vi "叶绿素a_获取温度和叶绿素值.vi"(8 "error in (no error)":errorcluster caption="错误输入（无错误）", 11 "MB session in":refnum<class "MB_Master.lvclass">) -> (0 "error out":errorcluster caption="错误输出", 2 "输出值":cluster{"温度测量值":sgl, "叶绿素测量值":sgl, "错误标志":u16} {"错误标志" items=["NO Error"=0, "刷子没到位"=255]}, 3 "MB session out":refnum<class "MB_Master.lvclass">)   [LabVIEW 2016, in "斯坦道多参数.lvlib"]
uses:
  <vilib>/Plasmionique/MB Master/MB_Master/MB_Master.lvclass
  <vilib>/Plasmionique/MB Master/MB Master.lvlib
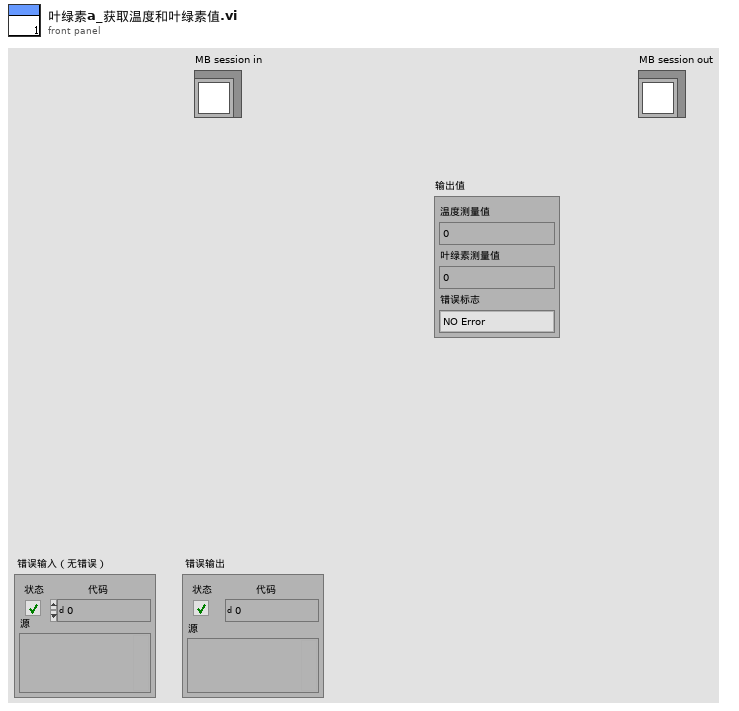
[diagram p1: front panel]
types:
  T1 = cluster{"pH":u32, "DO":u32, "Cond":u32, "Turb":u32, "叶绿素a":u32, "藻密度":u32, "ORP":u32}
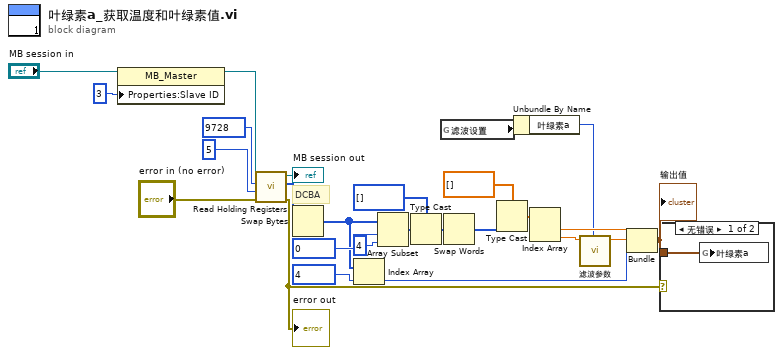
[diagram p0: block diagram]
diagram:
  # "DCBA"
  n1 = property class="MB_Master"(reference="MB session in", "Properties:Slave ID"=u16 3 ("y")) -> (reference out=w15:refnum<class "MB_Master.lvclass">)  [unwired: 1 in, 1 out]
  n2 = call <vilib>:"Read Holding Registers.vi"("error in (no error)"="error in (no error)", "quantity"=u16 5, "starting address"=u16 9728, "MB session in"=w15) -> ("error out"=w8:errorcluster, "Registers"=w11:u16[], "MB session out"=→"MB session out":refnum<class "MB_Master.lvclass">)  [unwired: 5 in]
  "error out" <- w8
  n3 = Swap Bytes(anything=w11) -> (byte swapped=w10:u16[])
  n4 = Index Array(array=w10, index=u16 4 ("starting address")) -> (element=w12:u16)
  n5 = Array Subset(array=w10, index=u16 0 ("starting address"), length=4 ("长度")) -> (w9:u16[])
  n6 = Type Cast(type=u32[] [] ("数组 2"), x=w9) -> (*(type *) &x=w21:u32[])
  n7 = global read "断电保存变量.vi" "滤波设置"() -> (w2:T1)
  n8 = Swap Words(1:w21) -> (0:w23:u32[])
  n9 = Type Cast(type=sgl[] [] ("数组 2"), x=w23) -> (*(type *) &x=w19:sgl[])
  n10 = Unbundle By Name(w2) -> ("叶绿素a"=w1:u32)
  n11 = Index Array(array=w19) -> (element #1=w18:sgl, element #2=w4:sgl)  [unwired: 2 in]
  n12 = call "滤波参数.vi"("滤波次数"=w1, "x"=w4) -> ("mode"=w3:dbl)  [unwired: 9 in]
  n13 = Bundle("数值"=w18, "mode"=w3, w12) -> (w7:cluster{"数值":sgl, "mode":dbl, u16})  [unwired: 1 in]
  "输出值" <- w7
  n14 = case shown="无错误" w8 {
    tunnel: w7 -> [w27 _]
    frame No Error {
      n15 = global write "禹山过程全局变量.vi" "叶绿素a"(w27) -> ()
    }
    frame Error {
    }
  }
